vi "SubVI_ReadTxt.vi"(8 "error in":errorcluster, 10 "Range Slide":cluster{dbl, dbl}={0.0, 1.0}, 11 "file path (use dialog)":path=path "D:/Desktop/A  2013-0104-1030-14.txt") -> (0 "error out":errorcluster, 1 "Data Array":dbl[][](array[numeric]), 2 "Title":string[](array[string]), 3 "path":path)   [LabVIEW 2011]
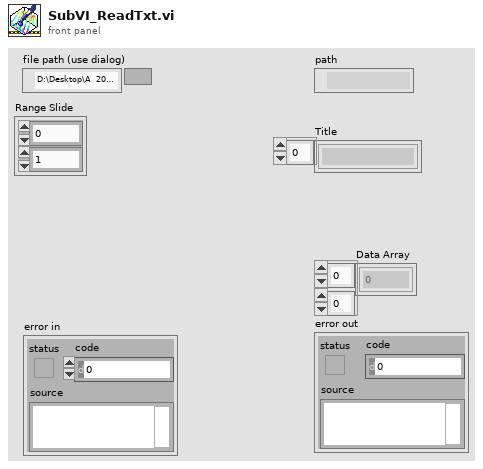
[diagram p1: front panel]
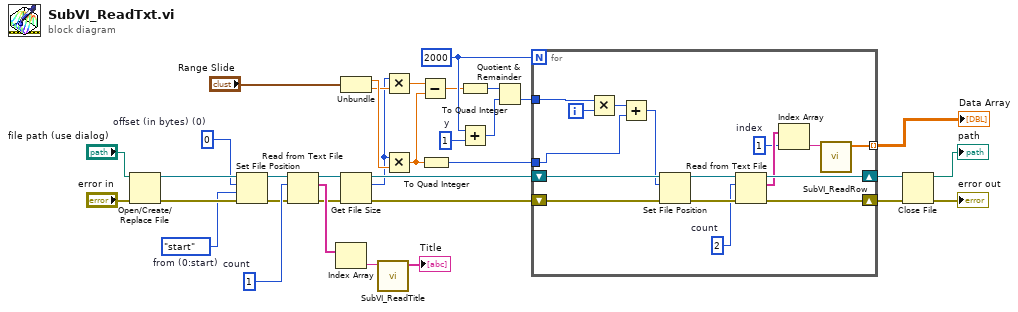
[diagram p0: block diagram]
diagram:
  w2 = enum16{"start", "end", "current"}."start"  # from (0:start)
  w3 = i64 0  # offset (in bytes) (0)
  w12 = 1  # count
  w27 = 1  # y
  w29 = 2000
  n1 = Open/Create/Replace File(file path (use dialog)="file path (use dialog)", error in="error in") -> (refnum out=w7:refnum<file>, error out=w4:errorcluster)  [unwired: 4 in, 1 out]
  n2 = Set File Position(offset (in bytes) (0)=w3, refnum=w7, from (0:start)=w2, error in=w4) -> (refnum out=w6:refnum<file>, error out=w5:errorcluster)
  n3 = Read from Text File(file (use dialog)=w6, count=w12, error in=w5) -> (refnum out=w9:refnum<file>, text=w13:string[], error out=w8:errorcluster)  [unwired: 1 in, 1 out]
  n4 = Index Array(array=w13) -> (element=w11:string)  [unwired: 1 in]
  n5 = Unbundle("Range Slide") -> (w21:dbl, w20:dbl)
  n6 = Get File Size(file=w9, error in=w8) -> (refnum out=w34:refnum<file>, size (in bytes)=w19:i64, 0:w33:errorcluster)
  n7 = call "SubVI_ReadTitle.vi"("String"=w11) -> ("Title"=→"Title":string[])  [unwired: 10 in]
  n8 = Multiply(x=w19, y=w20) -> (x*y=w18:dbl)
  n9 = Multiply(x=w19, y=w21) -> (x*y=w15:dbl)
  n10 = Subtract(x=w18, y=w15) -> (x-y=w17:dbl)
  n11 = To Quad Integer(1:w15) -> (0:w14:i64)
  n12 = To Quad Integer(1:w17) -> (0:w16:i64)
  n13 = Add(x=w29, y=w27) -> (x+y=w28:i32)
  n14 = Quotient & Remainder(x=w16, y=w28) -> (floor(x/y)=w26:i64)  [unwired: 1 out]
  n15 = for {
    N: w29 -> [_]
    shift-right: [w41] -> w31
    shift-left: w34 -> [w50]
    shift-right: [w40] -> w30
    shift-left: w33 -> [w49]
    tunnel: w26 -> [w45]
    tunnel: [w43] -> w1 mode=indexing
    tunnel: w14 -> [w35]
    i -> [w46]
    w37 = 1  # index
    w42 = 2  # count
    n16 = Multiply(x=w45, y=w46) -> (x*y=w44:i64)
    n17 = Add(x=w44, y=w35) -> (x+y=w36:i64)
    n18 = Set File Position(offset (in bytes) (0)=w36, refnum=w50, error in=w49) -> (refnum out=w48:refnum<file>, error out=w47:errorcluster)  [unwired: 1 in]
    n19 = Read from Text File(file (use dialog)=w48, count=w42, error in=w47) -> (refnum out=w41:refnum<file>, text=w39:string[], error out=w40:errorcluster)  [unwired: 1 in, 1 out]
    n20 = Index Array(array=w39, index=w37) -> (element=w38:string)
    n21 = call "SubVI_ReadRow.vi"("String"=w38) -> ("Row"=w43:dbl[])  [unwired: 10 in]
  }
  "Data Array" <- w1
  n22 = Close File(refnum=w31, error in=w30) -> (path=→"path":path, error out=→"error out":errorcluster)
